vi "Play Sound.vi"(8 "error in (no error)":errorcluster, 10 "Sound Type":string, 11 "Matlab Connection":refnum<k5>) -> (0 "error out":errorcluster, 2 "Return value I32":i32, 3 "connection ID out":refnum<k5>)   [LabVIEW 2014, in "Matlab API.lvlib"]
uses:
  Matlab API.lvlib
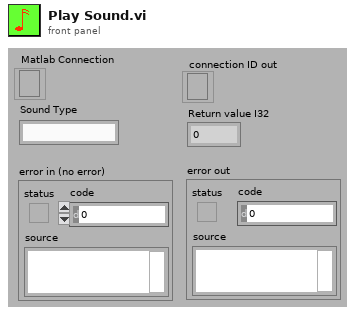
[diagram p1: front panel]
types:
  T1 = cluster{"Variable name":string, "Sound Type":string}
  T2 = cluster{"Variable name":string, "Sound Type":string}[]
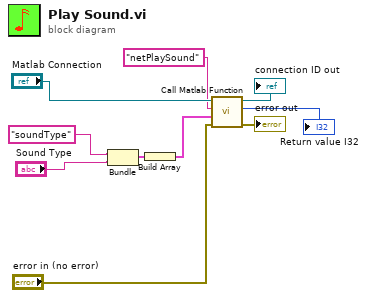
[diagram p0: block diagram]
diagram:
  n1 = Bundle("Variable name"="soundType", "Sound Type"="Sound Type") -> (w3:T1)  [unwired: 1 out]
  n2 = Build Array(w3) -> (w2:T2)
  n3 = call "Call Matlab Function.vi"("error in (no error)"="error in (no error)", "Matlab Param Array"=w2, "Function name"="netPlaySound", "TCP Network Connection Refnum"="Matlab Connection") -> ("error out"=→"error out":errorcluster, "Return value I32"=→"Return value I32":i32, "connection ID out"=→"connection ID out":refnum<k5>)  [unwired: 5 out]
